vi "Find First Digit.vi"(11 "String in":string) -> (3 "String out":string)   [LabVIEW 2022 SP3]
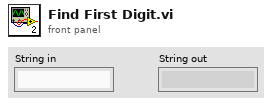
[diagram p1: front panel]
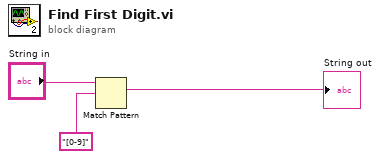
[diagram p0: block diagram]
diagram:
  n1 = Match Pattern(string="String in", regular expression="[0-9]" ("format string")) -> (match substring=→"String out":string)  [unwired: 1 in, 3 out]
